vi "Convert JSON Cluster to Runtime Cluster.vi"(8 "error in (no error)":errorcluster, 11 "Framework JSON Configuration":T13) -> (0 "error out":errorcluster, 3 "Framework Configuration":T1)   [LabVIEW 2017, in "DSF Core.lvlib" / "JSON Builder.lvclass"]
uses:
  JSON Builder.lvclass
  Typedefs/DSF Engine Framework JSON Configuration.ctl
  Typedefs/DSF Engine Plugin JSON Configuration.ctl
  Typedefs/DSF Timing Info.ctl
  Typedefs/DSF Engine Plugin Thread Configuration.ctl
  Typedefs/DSF Settings Info.ctl
  Typedefs/DSF Engine Transfer Group JSON Configuration.ctl
  Typedefs/DSF Engine Transfer JSON Configuration.ctl
  Typedefs/DSF Engine Channel JSON Configuration.ctl
  Typedefs/DSF Engine Framework Configuration.ctl
  Typedefs/DSF Engine Plugin Configuration.ctl
  Typedefs/DSF Engine Transfer Group Configuration.ctl
  Typedefs/DSF Direction.ctl
  Typedefs/DSF Engine Transfer Configuration.ctl
  Typedefs/DSF Byte Order.ctl
  Typedefs/DSF Engine Channel Configuration.ctl
  Typedefs/DSF Data Type.ctl
  Typedefs/DSF Timeout Behavior.ctl
  DSF Core.lvlib
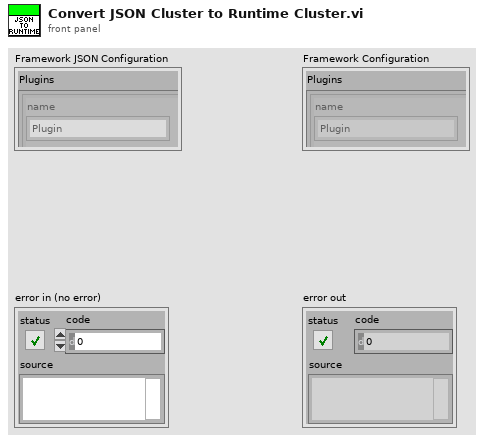
[diagram p1: front panel]
types:
  T1 = typedef "DSF Core.lvlib/DSF Engine Framework Configuration.ctl" = cluster{"Plugins":T2[]}
  T2 = typedef "DSF Core.lvlib/DSF Engine Plugin Configuration.ctl" = cluster{"name":string, "components":string[], "cycle timing":T3, "threads":T4[], "Transfer Groups":T6[], "settings":T5}
  T3 = typedef "DSF Core.lvlib/DSF Timing Info.ctl" = cluster{"priority":u64, "decimation":u64, "offset":u64}
  T4 = typedef "DSF Core.lvlib/DSF Engine Plugin Thread Configuration.ctl" = cluster{"buffer converter settings":T5, "transceiver settings":T5, "custom settings":T5, "processor":i32, "priority offset":i16}
  T5 = typedef "DSF Core.lvlib/DSF Settings Info.ctl" = cluster{"key":string, "value":string}[]
  T6 = typedef "DSF Core.lvlib/DSF Engine Transfer Group Configuration.ctl" = cluster{"name":string, "direction":T7, "cycle timing":T3, "thread index":i32, "settings":T5, "Transfers":T8[], "timeout behavior":T12}
  T7 = typedef "DSF Core.lvlib/DSF Direction.ctl" = enum8{"Tx", "Rx"}
  T8 = typedef "DSF Core.lvlib/DSF Engine Transfer Configuration.ctl" = cluster{"name":string, "byte order":T9, "settings":T5, "channels":T10[]}
  T9 = typedef "DSF Core.lvlib/DSF Byte Order.ctl" = enum8{"big-endian", "little-endian"}
  T10 = typedef "DSF Core.lvlib/DSF Engine Channel Configuration.ctl" = cluster{"string offset":u64, "string data type":T11, "engine data type":T11, "name":string, "settings":T5, "units":string}
  T11 = typedef "DSF Core.lvlib/DSF Data Type.ctl" = enum8{"Bool", "SGL", "DBL", "I8", "I16", "I32", "I64", "U8", "U16", "U32", "U64"}
  T12 = typedef "DSF Core.lvlib/DSF Timeout Behavior.ctl" = enum8{"Increment Late Count", "Throw Error"}
  T13 = typedef "DSF Core.lvlib/JSON Builder.lvclass/DSF Engine Framework JSON Configuration.ctl" = cluster{"Plugins":T14[]}
  T14 = typedef "DSF Core.lvlib/JSON Builder.lvclass/DSF Engine Plugin JSON Configuration.ctl" = cluster{"name":string, "components":string[], "cycle timing":T3, "threads":T4[], "Transfer Groups":T15[], "settings":T5}
  T15 = typedef "DSF Core.lvlib/JSON Builder.lvclass/DSF Engine Transfer Group JSON Configuration.ctl" = cluster{"name":string, "direction":u8, "cycle timing":T3, "thread index":i32, "settings":T5, "Transfers":T16[], "timeout behavior":u8}
  T16 = typedef "DSF Core.lvlib/JSON Builder.lvclass/DSF Engine Transfer JSON Configuration.ctl" = cluster{"name":string, "byte order":u8, "settings":T5, "channels":T17[]}
  T17 = typedef "DSF Core.lvlib/JSON Builder.lvclass/DSF Engine Channel JSON Configuration.ctl" = cluster{"string offset":u64, "string data type":u8, "engine data type":u8, "name":string, "settings":T5, "units":string}
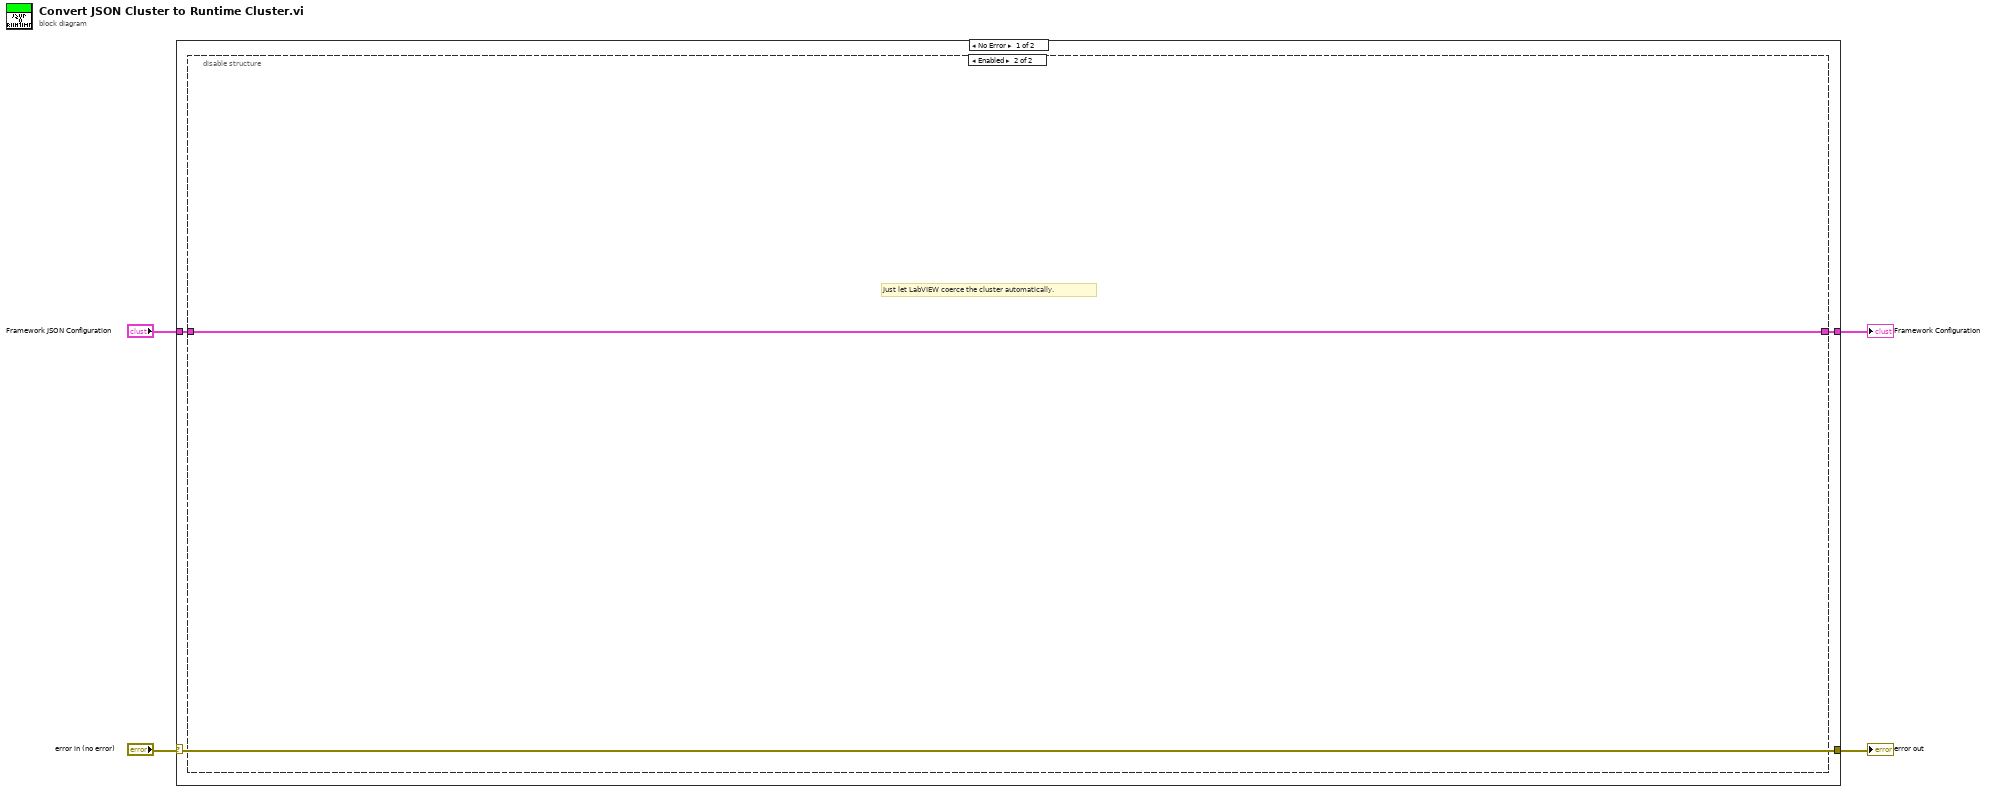
[diagram p0: block diagram]
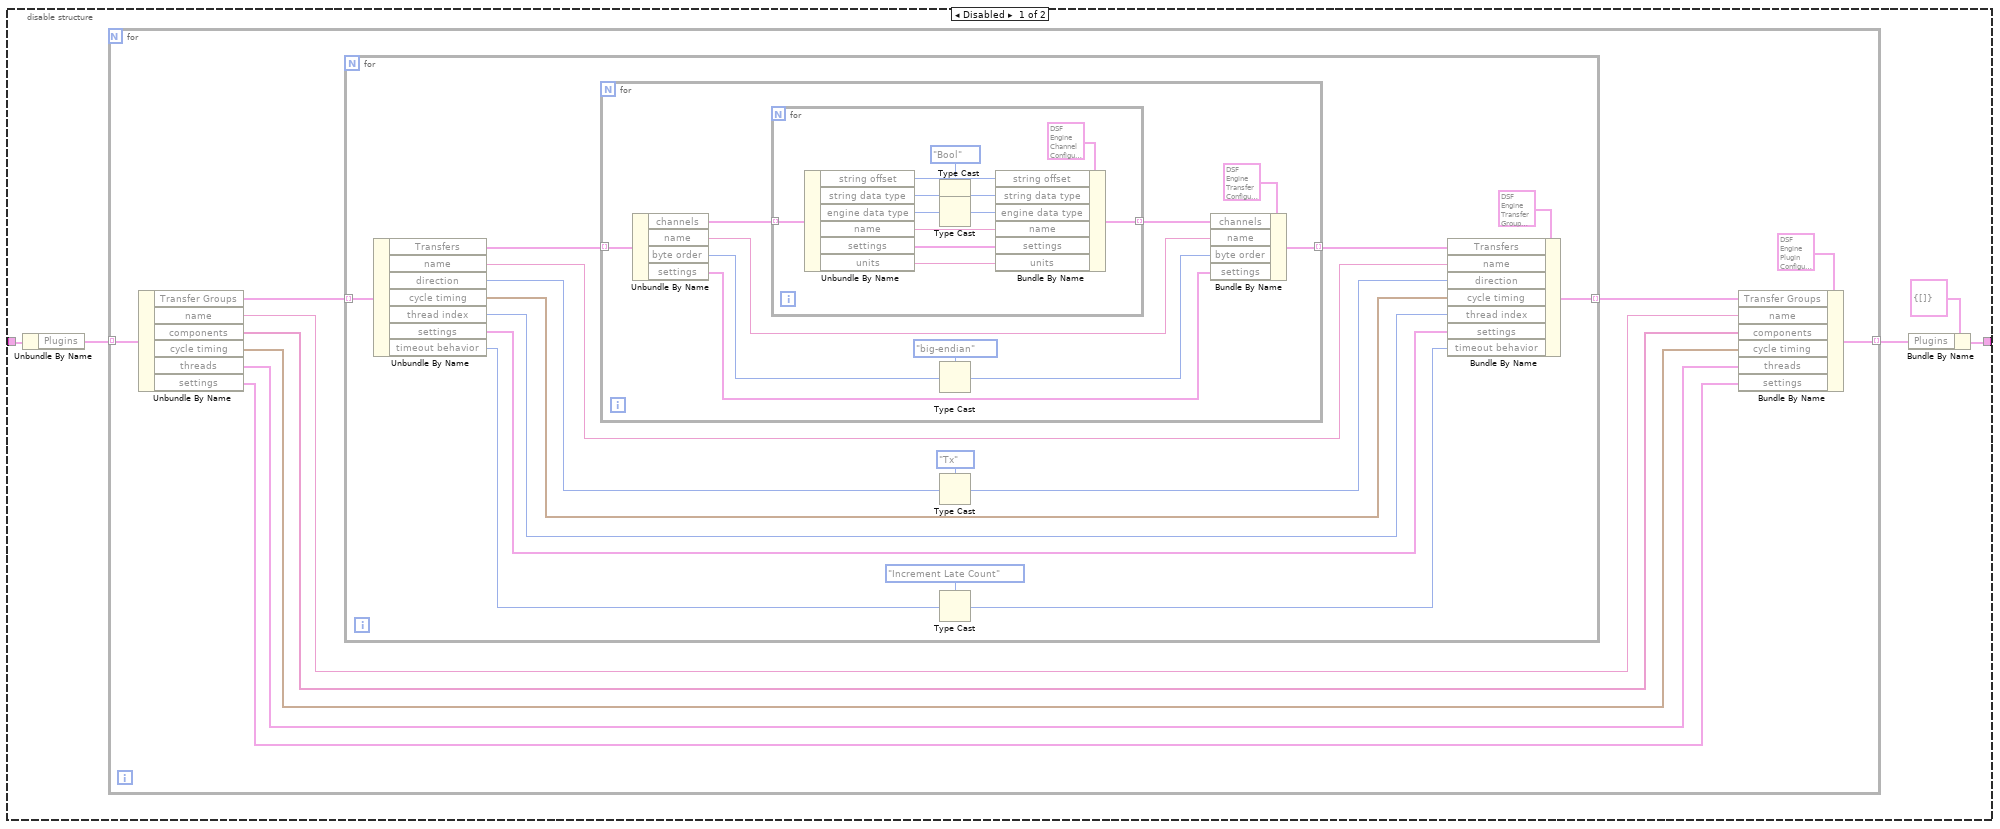
[diagram p2: hidden frame]
diagram:
  n1 = case shown="No Error" "error in (no error)" {
    selector: "error in (no error)" -> [w5 w61]
    tunnel: [w7 _] -> w1
    tunnel: "Framework JSON Configuration" -> [w6 _]
    tunnel: [w5 w61] -> w3
    frame No Error {
      n2 = disable-structure shown="Enabled" {
        disable-tunnel: [w10 w60] -> w7
        disable-tunnel: w6 -> [w8 w60]
        frame Disabled {
          n3 = Unbundle By Name(w8) -> ("Plugins"=w11:T14[])
          n4 = for {
            tunnel: w11 -> [w22] mode=indexing
            tunnel: [w13] -> w12 mode=indexing
            n5 = Unbundle By Name(w22) -> ("Transfer Groups"=w21:T15[], "name"=w14:string, "components"=w18:string[], "cycle timing"=w17:T3, "threads"=w16:T4[], "settings"=w15:T5)
            n6 = for {
              tunnel: w21 -> [w37] mode=indexing
              tunnel: [w29] -> w19 mode=indexing
              n7 = Unbundle By Name(w37) -> ("Transfers"=w36:T16[], "name"=w33:string, "direction"=w28:u8, "cycle timing"=w32:T3, "thread index"=w31:i32, "settings"=w30:T5, "timeout behavior"=w25:u8)
              n8 = for {
                tunnel: w36 -> [w47] mode=indexing
                tunnel: [w41] -> w34 mode=indexing
                n9 = Unbundle By Name(w47) -> ("channels"=w46:T17[], "name"=w43:string, "byte order"=w39:u8, "settings"=w42:T5)
                n10 = for {
                  tunnel: w46 -> [w59] mode=indexing
                  tunnel: [w53] -> w44 mode=indexing
                  w50 = DSF_Data_Type."Bool" ("string data type")
                  n11 = Unbundle By Name(w59) -> ("string offset"=w54:u64, "string data type"=w52:u8, "engine data type"=w51:u8, "name"=w55:string, "settings"=w56:T5, "units"=w57:string)
                  n12 = Type Cast(type=w50, x=w52) -> (*(type *) &x=w49:T11)
                  n13 = Type Cast(type=w50, x=w51) -> (*(type *) &x=w48:T11)
                  n14 = Bundle By Name(cluster=T10 {"string offset"=0, "string data type"=enum."DBL", "engine data type"=enum."DBL", "name"="Channel", "settings"=[], "units"="V"} ("channel configuration"), "string offset"=w54, "string data type"=w49, "engine data type"=w48, "name"=w55, "settings"=w56, "units"=w57) -> (w53:T10)
                }
                n15 = Type Cast(type=DSF_Byte_Order."big-endian" ("byte order"), x=w39) -> (*(type *) &x=w38:T9)
                n16 = Bundle By Name(cluster=T8 {"name"="Transfer", "byte order"=enum."big-endian", "settings"=[], "channels"=[]} ("Transfer Configuration"), "channels"=w44, "name"=w43, "byte order"=w38, "settings"=w42) -> (w41:T8)
              }
              n17 = Type Cast(type=DSF_Direction."Tx" ("direction"), x=w28) -> (*(type *) &x=w27:T7)
              n18 = Type Cast(type=DSF_Timeout_Behavior."Increment Late Count" ("timeout behavior"), x=w25) -> (*(type *) &x=w24:T12)
              n19 = Bundle By Name(cluster=T6 {"name"="Group", "direction"=enum."Tx", "cycle timing"={"priority"=100, "decimation"=1, "offset"=0}, "thread index"=-1, "settings"=[], "Transfers"=[], "timeout behavior"=enum."Increment Late Count"} ("Transfer Group Configuration"), "Transfers"=w34, "name"=w33, "direction"=w27, "cycle timing"=w32, "thread index"=w31, "settings"=w30, "timeout behavior"=w24) -> (w29:T6)
            }
            n20 = Bundle By Name(cluster=T2 {"name"="Plugin", "components"=[], "cycle timing"={"priority"=10000, "decimation"=1, "offset"=0}, "threads"=[], "Transfer Groups"=[], "settings"=[]} ("Plugin Configuration"), "Transfer Groups"=w19, "name"=w14, "components"=w18, "cycle timing"=w17, "threads"=w16, "settings"=w15) -> (w13:T2)
          }
          n21 = Bundle By Name(cluster=T1 {"Plugins"=[]} ("Framework Configuration"), "Plugins"=w12) -> (w10:T1)
        }
        frame Enabled {
          # "Just let LabVIEW coerce the cluster automatically."
        }
      }
    }
    frame Error {
    }
  }
  "Framework Configuration" <- w1
  "error out" <- w3
